vi "TEST_CONFIGURABLE SMO.vi"() -> ()   [LabVIEW 2013]
uses:
  Config--cluster.ctl
  <vilib>/LabVIEW Open Source/Configuration Manager/Manager/ConfigManager.lvclass
  <vilib>/LabVIEW Open Source/Configuration Manager/Manager/ConfigManager.lvclass/ConfigManager.ctl
  <vilib>/LabVIEW Open Source/Configuration Manager/Serializer/Serializer.lvclass
  <vilib>/LabVIEW Open Source/Configuration Manager/Encoding/Encoding.lvclass
  <vilib>/LabVIEW Open Source/Configuration Manager/Encryption/Encryption.lvclass
  src/SMO/Typedefs/SMOState --Enum.ctl
  <vilib>/LabVIEW Open Source/Configuration Manager/Manager/Read Serializer.vi
  <vilib>/LabVIEW Open Source/Configuration Manager/Manager/Read Encoding.vi
  <vilib>/LabVIEW Open Source/Configuration Manager/Manager/Read Encryption.vi
  <vilib>/Utility/VariantDataType/GetTypeInfo.vi
  SMO.Configurable.lvclass
  src/SMO/SMO.lvclass
  <vilib>/LabVIEW Open Source/Configuration Manager/Cache/ConfigManager.Cache.lvclass
panel:
  out "keys changed":string[](array[string])
  out "error out":errorcluster
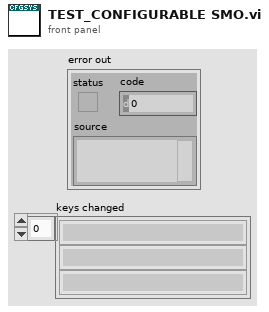
[diagram p1: front panel]
types:
  T1 = typedef "SMO.Configurable.lvclass/Config--cluster.ctl" = cluster{"timeout":i32, "run":bool}
  T2 = typedef "SMO.lvclass/Public Events.ctl" = cluster{"Error":refnum<user-event>, "State":refnum<user-event>, "Reserve State":refnum<user-event>}
  T3 = typedef "SMO.lvclass/SMOState --Enum.ctl" = enum16{"unknown", "Created", "Started", "Stopped"}
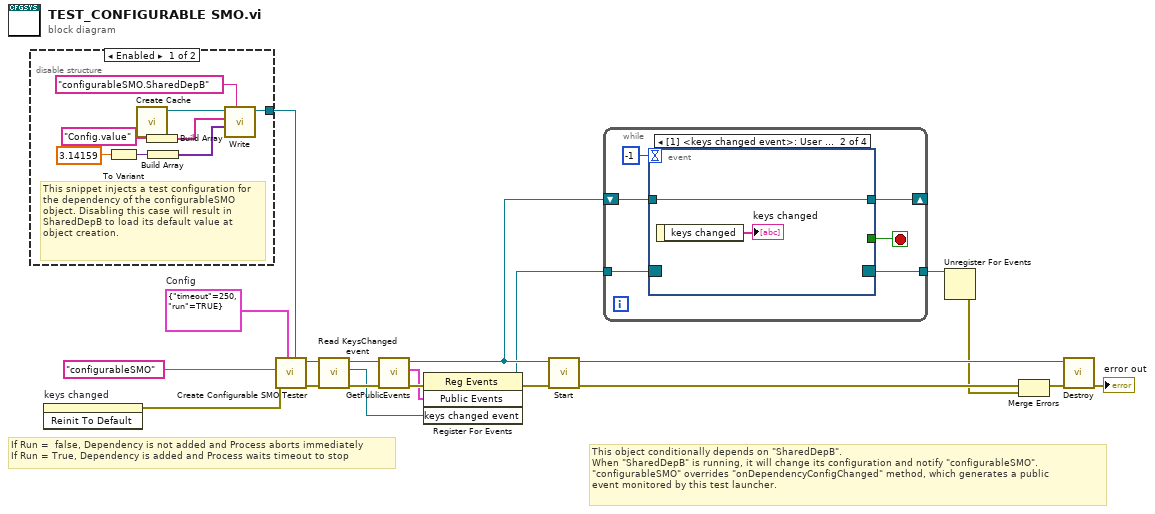
[diagram p0: block diagram]
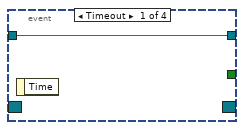
[diagram p3: hidden frame]
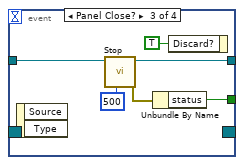
[diagram p4: hidden frame]
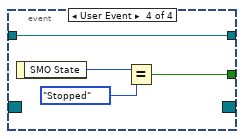
[diagram p5: hidden frame]
diagram:
  w19 = T1 {"timeout"=250, "run"=TRUE}  # Config
  # "This object conditionally depends on \"SharedDepB\".\nWhen \"SharedDepB\" is running, it will change its configuration and notify \"configurableSMO\".\n\"configurableSMO\" overrides \"onDependencyConfigChanged\" method, which generates a public\nevent monitored by this test launcher."
  # "If Run =  false, Dependency is not added and Process aborts immediately\nIf Run = True, Dependency is added and Process waits timeout to stop"
  n1 = disable-structure shown="Enabled" {
    disable-tunnel: [w21 _] -> w7
    frame Enabled {
      # "This snippet injects a test configuration for the dependency of the configurableSMO object. Disabling this case will result in SharedDepB to load its default value at object creation."
      n2 = To Variant(anything=3.14159) -> (Variant=w24:variant)
      n3 = call <vilib>:"Create Cache.vi"() -> ("ConfigManager.Cache"=w28:refnum<class "ConfigManager.Cache.lvclass">)  [unwired: 11 in]
      n4 = Build Array("Config.value" ("Name")) -> (w25:string[])
      n5 = Build Array(w24) -> (w23:variant[])
      n6 = call <vilib>:"Write.vi"("Qualified Name"="configurableSMO.SharedDepB", "Values"=w23, "keys"=w25, "ConfigManager in"=w28) -> ("ConfigManager out"=w21:refnum<class "ConfigManager.Cache.lvclass">)  [unwired: 5 in, 2 out]
    }
    frame Disabled {
    }
  }
  n7 = invoke on="keys changed" class="Arr (strict)" method="Reinit To Default"() -> (error out=w1:errorcluster)  [unwired: 3 in, 2 out]
  n8 = call "Create Configurable SMO Tester.vi"("ConfigManager"=w7, "Config"=w19, "error in (no error)"=w1, "Subsystem Name (optional)"="configurableSMO") -> ("error out"=w4:errorcluster, "SMO.Configurable out"=w6:refnum<class "SMO.Configurable.lvclass">)  [unwired: 5 in, 1 out]
  n9 = call "Read KeysChanged event.vi"("error in (no error)"=w4, "SMO.Configurable in"=w6) -> ("error out"=w3:errorcluster, "keys changed event"=w2:refnum<user-event>, "SMO.Configurable out"=w5:refnum<class "SMO.Configurable.lvclass">)  [unwired: 7 in]
  n10 = call "GetPublicEvents.vi"("error in (no error)"=w3, "SMO"=w5) -> ("error out"=w15:errorcluster, "Public Events"=w14:T2, "SMO out"=w12:refnum<class "SMO.Configurable.lvclass">)  [unwired: 7 in]
  n11 = register-events(error in=w15, w14, w2) -> (reference out=w11:refnum<event-registration>, error out=w13:errorcluster)  [unwired: 1 in]
  n12 = call "Start.vi"("error in (no error)"=w13, "SMO"=w12) -> ("error out"=w16:errorcluster, "SMO out"=w18:refnum<class "SMO.Configurable.lvclass">)  [unwired: 8 in]
  n13 = while {
    shift-right: [w30] -> _
    shift-left: w12 -> [w33]
    tunnel: w11 -> [w32]
    tunnel: [w31] -> w10
    stop <- w29 stop-if-true
    n14 = event shown="[1] <keys changed event>: User Event" {
      selector: w32 -> [_ _ _ _]
      dyn-events: [_ _ _ _] -> w31
      timeout: -1 -> [_ _ _ _]
      tunnel: w33 -> [w35 w37 w42 w47]
      tunnel: [w35 w37 w41 w47] -> w30
      tunnel: [_ _ w39 w44] -> w29
      event Timeout {
        n15 = event-data() -> ()  [unwired: 1 in, 1 out]
      }
      event User Event {
        n16 = event-data() -> ("keys changed"=→"keys changed":string[])  [unwired: 1 in]
      }
      event Panel Close? {
        n17 = event-data() -> ()  [unwired: 1 in, 2 out]
        n18 = call "Stop.vi"("timeout in ms (-1)"=500, "SMO"=w42) -> ("error out"=w40:errorcluster, "SMO out"=w41:refnum<class "SMO.Configurable.lvclass">)  [unwired: 8 in]
        n19 = Unbundle By Name(w40) -> ("status"=w39:bool)
        n20 = event-data("Discard?"=TRUE) -> ()  [unwired: 1 in, 1 out]
      }
      event User Event {
        n21 = event-data() -> ("SMO State"=w46:T3)  [unwired: 1 in]
        n22 = Equal?(x=w46, y=SMOState_--Enum."Stopped") -> (x = y?=w44:bool)
      }
    }
  }
  n23 = Unregister For Events(event registration refnum=w10) -> (error out=w9:errorcluster)  [unwired: 1 in]
  n24 = Merge Errors(w16, w9) -> (w17:errorcluster)
  n25 = call "Destroy.vi"("error in (no error)"=w17, "SMO"=w18) -> ("error out"=→"error out":errorcluster)  [unwired: 9 in]
